vi "CalcPodOutputVectors.vi"(9 "Linear Magnitude value, [-1,1]":dbl, 10 "Direction value, [-pi,pi]":dbl, 11 "Rotation value, [-1,1]":dbl) -> (3 "Pod Output Vectors":cluster{"Magnitude":dbl, "Direction":dbl}[](array[cluster]))   [LabVIEW 2014]
uses:
  Variables/Physical data.vi
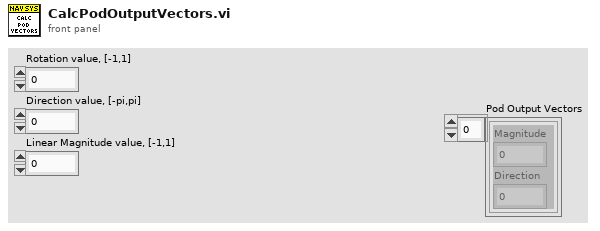
[diagram p1: front panel]
types:
  T1 = typedef "NI_Matrix.lvlib/RealMatrix.ctl" = dbl[][]
  T2 = cluster{"All Pod State Data":cluster{"Drive":cluster{"Drive Motor Output":dbl, "Wheel RPM":dbl, "Linear speed":dbl, "Linear acceleration":dbl, "Encoder Output":dbl, "Vmot":dbl, "Imot":dbl, "Torque":dbl, "Angular Momentum":dbl}, "Turret":cluster{"Turret Motor Output":dbl, "Turret Angle":dbl, "Turret velocity":dbl, "Turret acceleration":dbl, "Encoder Output":dbl, "Vmot":dbl, "Imot":dbl, "Torque":dbl, "Angular Momentum":dbl}, "Pod position (RCS)":cluster{"X":dbl, "Y":dbl, "Z":dbl}}[], "Global Robot Data":cluster{"Position Data":cluster{"Robot Position":cluster{"X":dbl, "Y":dbl, "Z":dbl}, "Robot Velocity":cluster{"X":dbl, "Y":dbl, "Z":dbl}, "Robot Acceleration":cluster{"X":dbl, "Y":dbl, "Z":dbl}}, "Rotation Data":cluster{"Angular Position":cluster{"X":dbl, "Y":dbl, "Z":dbl}, "Angular Velocity":cluster{"X":dbl, "Y":dbl, "Z":dbl}, "Angular Acceleration":cluster{"X":dbl, "Y":dbl, "Z":dbl}}}, "Inertial Characteristics":cluster{"Center of Mass (RCS)":cluster{"X":dbl, "Y":dbl, "Z":dbl}, "Mass Elements":cluster{"X":dbl, "Y":dbl, "Z":dbl, "Mass":dbl, "Name":string}[], "Center of Rotation (RCS)":cluster{"X":dbl, "Y":dbl, "Z":dbl}, "Tensor of Inertia":T1}}
  T3 = cluster{"PodConfigurations":cluster{"Drive":cluster{"Encoder":cluster{"CPft":dbl, "Location":string, "RIO_PinA":i32, "RIO_PinB":i32, "Invert?":bool}, "Motor":cluster{"PID":cluster{"P":dbl, "I":dbl, "D":dbl}, "CANorPWM Channel":i32, "Invert?":bool, "IsCanSRX?":bool, "Output":cluster{"Max":dbl, "Min":dbl}}}, "Turret":cluster{"Encoder":cluster{"ZeroPosVolts":dbl, "Location":string, "RIO_AnalogChannel":i32, "Invert?":bool}, "Motor":cluster{"PID":cluster{"P":dbl, "I":dbl, "D":dbl}, "CANorPWM Channel":i32, "Invert?":bool, "IsCanSRX?":bool, "Output":cluster{"Max":dbl, "Min":dbl}}}, "Misc":cluster{"Pod_Pos":cluster{"X":dbl, "Y":dbl}, "PDP_Channels":cluster{"Drive":i32, "Turret":i32}}}[], "General Configuration":cluster{"Pod Count":i32, "PDP CAN ID":i32, "PCM CAN ID":i32, "BaseRobotMass":dbl}}
  T4 = cluster{"Drive":cluster{"Encoder":cluster{"CPft":dbl, "Location":string, "RIO_PinA":i32, "RIO_PinB":i32, "Invert?":bool}, "Motor":cluster{"PID":cluster{"P":dbl, "I":dbl, "D":dbl}, "CANorPWM Channel":i32, "Invert?":bool, "IsCanSRX?":bool, "Output":cluster{"Max":dbl, "Min":dbl}}}, "Turret":cluster{"Encoder":cluster{"ZeroPosVolts":dbl, "Location":string, "RIO_AnalogChannel":i32, "Invert?":bool}, "Motor":cluster{"PID":cluster{"P":dbl, "I":dbl, "D":dbl}, "CANorPWM Channel":i32, "Invert?":bool, "IsCanSRX?":bool, "Output":cluster{"Max":dbl, "Min":dbl}}}, "Misc":cluster{"Pod_Pos":cluster{"X":dbl, "Y":dbl}, "PDP_Channels":cluster{"Drive":i32, "Turret":i32}}}[]
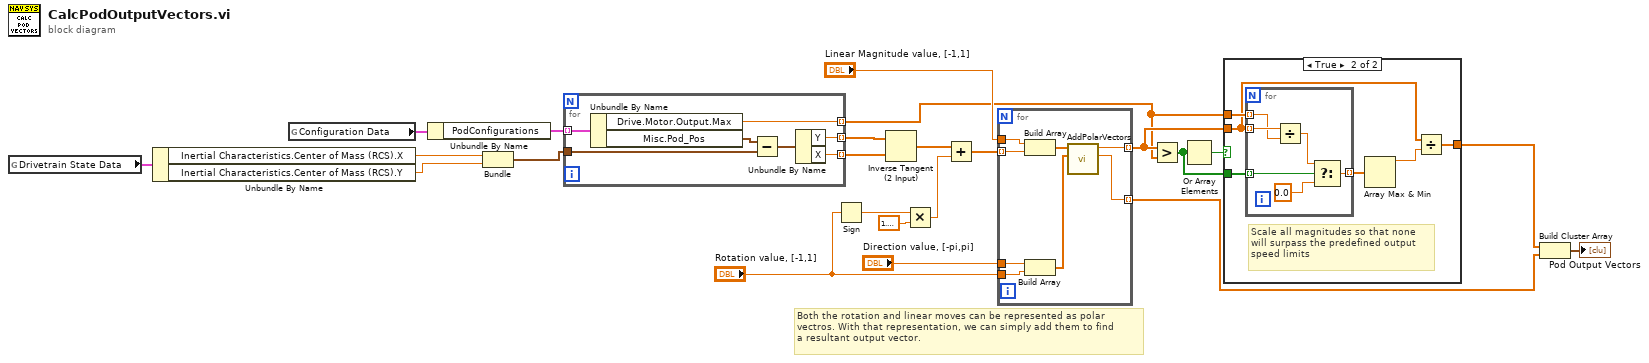
[diagram p0: block diagram]
diagram:
  # "Both the rotation and linear moves can be represented as polar\nvectros. With that representation, we can simply add them to find\na resultant output vector."
  n1 = global read "Physical data.vi" "Drivetrain State Data"() -> (w13:T2)
  n2 = Unbundle By Name(w13) -> ("Inertial Characteristics.Center of Mass (RCS).X"=w16:dbl, "Inertial Characteristics.Center of Mass (RCS).Y"=w15:dbl)
  n3 = global read "Physical data.vi" "Configuration Data"() -> (w12:T3)
  n4 = Unbundle By Name(w12) -> ("PodConfigurations"=w14:T4)
  n5 = Bundle("X"=w16, "Y"=w15) -> (w17:cluster{"X":dbl, "Y":dbl})  [unwired: 1 in]
  n6 = for {
    tunnel: w14 -> [w30] mode=indexing
    tunnel: w17 -> [w28]
    tunnel: [w26] -> w18 mode=indexing
    tunnel: [w25] -> w19 mode=indexing
    tunnel: [w24] -> w4 mode=indexing
    n7 = Unbundle By Name(w30) -> ("Drive.Motor.Output.Max"=w24:dbl, "Misc.Pod_Pos"=w29:cluster{"X":dbl, "Y":dbl})
    n8 = Subtract(x=w29, y=w28) -> (x-y=w27:cluster{"X":dbl, "Y":dbl})
    n9 = Unbundle By Name(w27) -> ("Y"=w26:dbl, "X"=w25:dbl)
  }
  n10 = Sign(1:"Rotation value, [-1,1]") -> (0:w20:dbl)
  n11 = Inverse Tangent (2 Input)(1:w19, 2:w18) -> (0:w22:dbl[])
  n12 = Multiply(x=w20, y=1.5707963267948966) -> (x*y=w23:dbl)
  n13 = Add(x=w22, y=w23) -> (x+y=w11:dbl[])
  n14 = for {
    tunnel: w11 -> [w37] mode=indexing
    tunnel: "Linear Magnitude value, [-1,1]" -> [w38]
    tunnel: "Direction value, [-pi,pi]" -> [w36]
    tunnel: "Rotation value, [-1,1]" -> [w35]
    tunnel: [w32] -> w6 mode=indexing
    tunnel: [w31] -> w2 mode=indexing
    n15 = Build Array(w38, w37) -> (w34:dbl[])
    n16 = Build Array(w36, w35) -> (w33:dbl[])
    n17 = call "AddPolarVectors.vi"("Angle1"=w33, "Magnitude"=w34) -> ("New Angle1"=w31:dbl, "New Magnitude"=w32:dbl)  [unwired: 7 in, 1 out]
  }
  n18 = Greater?(x=w6, y=w4) -> (0:w5:bool[])
  n19 = Or Array Elements(Boolean array=w5) -> (logical OR=w7:bool)
  n20 = case shown="True" w7 {
    tunnel: w6 -> [w39 w41]
    tunnel: w4 -> [_ w45]
    tunnel: w5 -> [_ w44]
    tunnel: [w39 w40] -> w3
    frame False {
    }
    frame True {
      # "Scale all magnitudes so that none\nwill surpass the predefined output \nspeed limits"
      n21 = for {
        tunnel: w45 -> [w50] mode=indexing
        tunnel: w41 -> [w51] mode=indexing
        tunnel: w44 -> [w49] mode=indexing
        tunnel: [w46] -> w43 mode=indexing
        n22 = Divide(x=w51, y=w50) -> (x/y=w48:dbl)
        n23 = Select(t=w48, s=w49, f=0.0) -> (s? t:f=w46:dbl)
      }
      n24 = Array Max & Min(array=w43) -> (max value=w42:dbl)  [unwired: 3 out]
      n25 = Divide(x=w41, y=w42) -> (x/y=w40:dbl[])
    }
  }
  n26 = Build Cluster Array(w3, w2) -> (→"Pod Output Vectors":cluster{"New Magnitude":dbl, "New Angle1":dbl}[])
